vi "procesare imagine.vi"(11 "image data":T1) -> (0 "image array":sgl[](array[numeric]), 3 "image 28x28":sgl[][](graph))   [LabVIEW 2024]
uses:
  <vilib>/picture/picture.llb/imagedata.ctl
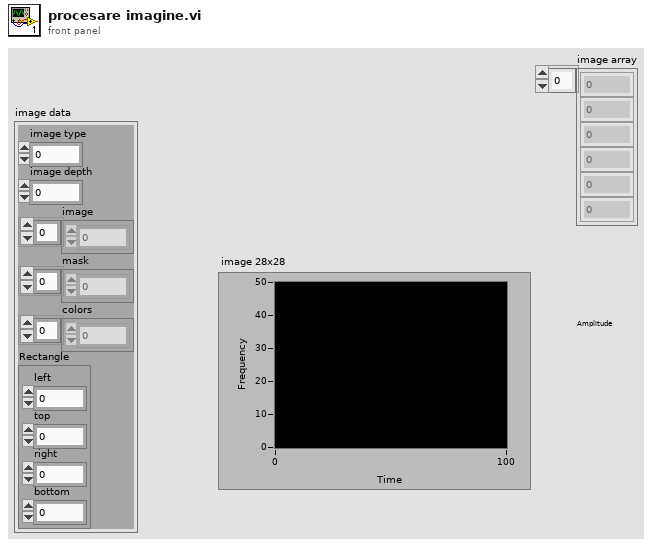
[diagram p1: front panel]
types:
  T1 = typedef "imagedata.ctl" = cluster{"image type":i32, "image depth":i32, "image":u8[], "mask":u8[], "colors":u32[], "Rectangle":cluster{"left":i16, "top":i16, "right":i16, "bottom":i16}}
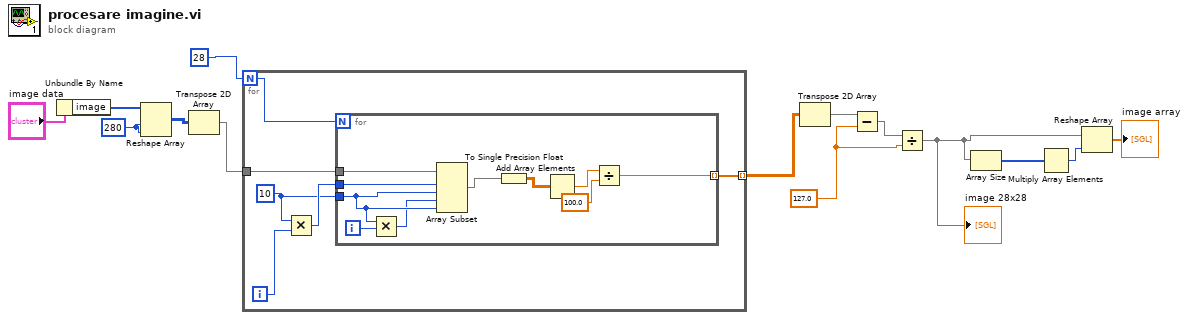
[diagram p0: block diagram]
diagram:
  w5 = sgl 127.0 ("y")
  w11 = 280 ("dimension size")
  n1 = Unbundle By Name("image data") -> ("image"=w13:u8[])
  n2 = Reshape Array(w13, w11, w11) -> (w12:u8[][])
  n3 = Transpose 2D Array(2D array=w12) -> (transposed array=w9:u8[][])
  n4 = for {
    N: 28 -> [w20]
    tunnel: w9 -> [w18]
    tunnel: [w15] -> w8 mode=indexing
    i -> [w19]
    w16 = 10
    n5 = Multiply(x=w16, y=w19) -> (x*y=w17:i32)
    n6 = for {
      N: w20 -> [_]
      tunnel: w18 -> [w30]
      tunnel: w17 -> [w29]
      tunnel: w16 -> [w27]
      tunnel: [w21] -> w15 mode=indexing
      i -> [w28]
      n7 = Multiply(x=w27, y=w28) -> (x*y=w26:i32)
      n8 = Array Subset(array=w30, index (row)=w29, length (row)=w27, index (col)=w26, length (col)=w27) -> (w25:u8[][])
      n9 = To Single Precision Float(number=w25) -> (single precision float=w24:sgl[][])
      n10 = Add Array Elements(numeric array=w24) -> (sum=w23:sgl)
      n11 = Divide(x=w23, y=sgl 100.0) -> (x/y=w21:sgl)
    }
  }
  n12 = Transpose 2D Array(2D array=w8) -> (transposed array=w7:sgl[][])
  n13 = Subtract(x=w7, y=w5) -> (x-y=w6:sgl[][])
  n14 = Divide(x=w6, y=w5) -> (x/y=w1:sgl[][])
  "image 28x28" <- w1
  n15 = Array Size(array=w1) -> (size(s)=w4:i32[])
  n16 = Multiply Array Elements(1:w4) -> (0:w3:i32)
  n17 = Reshape Array(w1, w3) -> (→"image array":sgl[])
